vi "Overlay Results.vi"(5 "Name":string, 7 "Overlay Setup":T1, 8 "error in (no error)":errorcluster, 9 "Matches (pixels)":T2(array[cluster]) {"Bounding Box"."y" format="%.2f"; "Bounding Box"."x" format="%.2f"; "Position"."y" format="%.2f"; "Position"."x" format="%.2f"; "Score" format="%.2f"; "Scale" format="%.2f"; "Angle" format="%.2f"}, 10 "Search Area":T3 {"Contours"."Type" items=["No Selection", "Point", "Line", "Rectangle", "Oval", "Polygon", "Free", "Annulus", "Unused2", "Unused3", "Broken Line", "Free Hand Line", "Rotated Rectangle"]}, 11 "Image In":T4) -> (0 "error out":errorcluster, 2 "Elapsed Time (ms)":u32, 3 "Image Out":T4)   [LabVIEW 2017]
uses:
  <vilib>/vision/Image Controls.llb/IMAQ Image.ctl
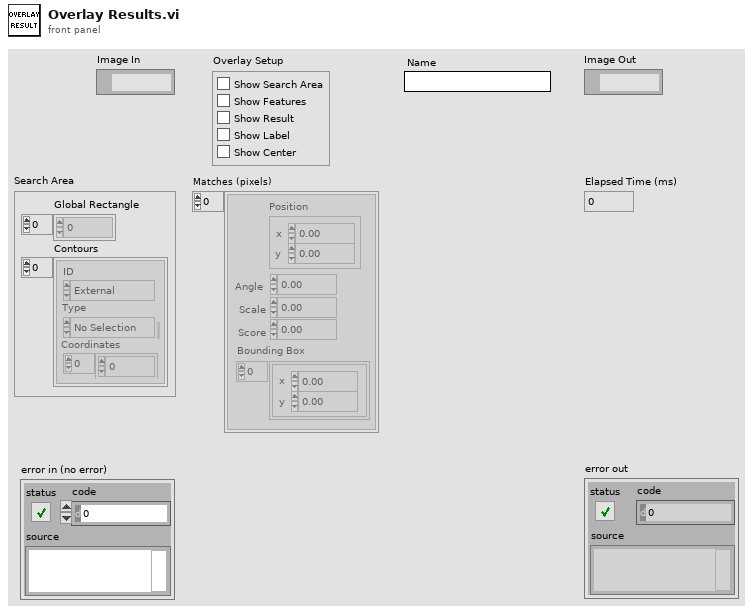
[diagram p1: front panel]
types:
  T1 = cluster{"Show Search Area":bool, "Show Features":bool, "Show Result":bool, "Show Label":bool, "Show Center":bool}
  T2 = cluster{"Position":cluster{"x":sgl, "y":sgl}, "Angle":sgl, "Scale":sgl, "Score":sgl, "Bounding Box":cluster{"x":sgl, "y":sgl}[]}[]
  T3 = cluster{"Global Rectangle":i32[], "Contours":cluster{"ID":enum32{"External", "Internal"}, "Type":u32, "Coordinates":i32[]}[]}
  T4 = typedef "IMAQ Image.ctl" = refnum<image>
  T5 = cluster{"Image":T4, "Search Area":cluster{"Global Rectangle":i32[], "Contours":cluster{"ID":enum32{"External", "Internal"}, "Type":u32, "Coordinates":i32[]}[]}, "Matches (pixels)":cluster{"Position":cluster{"x":sgl, "y":sgl}, "Angle":sgl, "Scale":sgl, "Score":sgl, "Bounding Box":cluster{"x":sgl, "y":sgl}[]}[], "Setup":cluster{"Show Search Area":bool, "Show Features":bool, "Show Result":bool, "Show Label":bool, "Show Center":bool}, "start time":u32, "Name":string}
  T6 = cluster{"Desired Font (Application)":enum16{"User-specified Font", "Application Font", "System Font", "Dialog Font"}, "[User-specified Font]":cluster{"Font Name":string, "Size":i16, "Strikeout?":bool, "Italic?":bool, "Underline?":bool, "Outline?":bool, "Shadow?":bool, "Bold?":bool, "Rotation Angle":dbl}, "Horizontal Alignment":i16, "Vertical Alignment":i16}
  T7 = cluster{"ID":enum32{"External", "Internal"}, "Type":u32, "Coordinates":i32[]}[]
  T8 = cluster{"ID":enum32{"External", "Internal"}, "Type":u32, "Coordinates":i32[]}
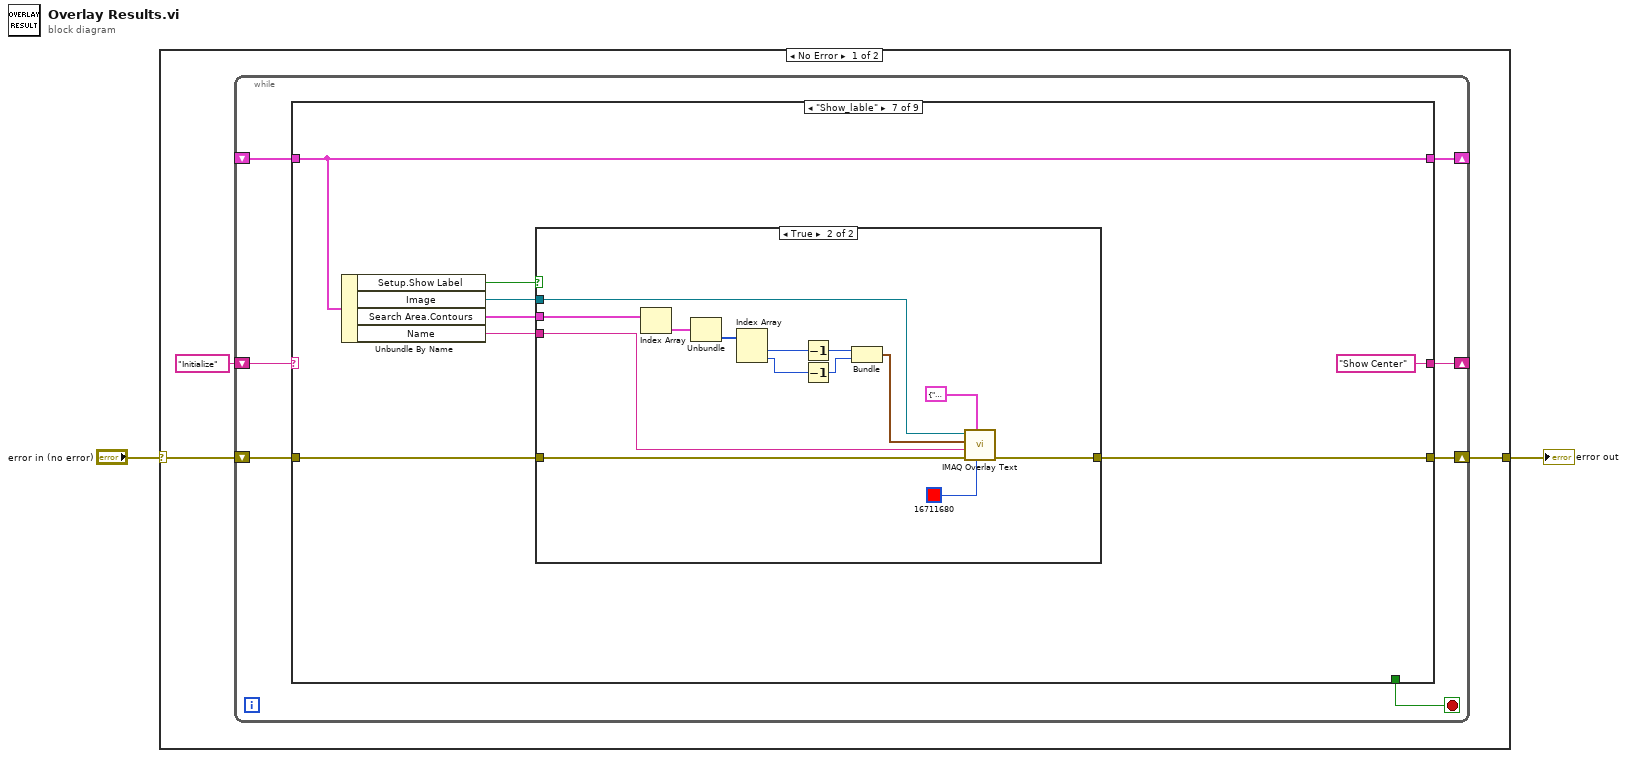
[diagram p0: block diagram]
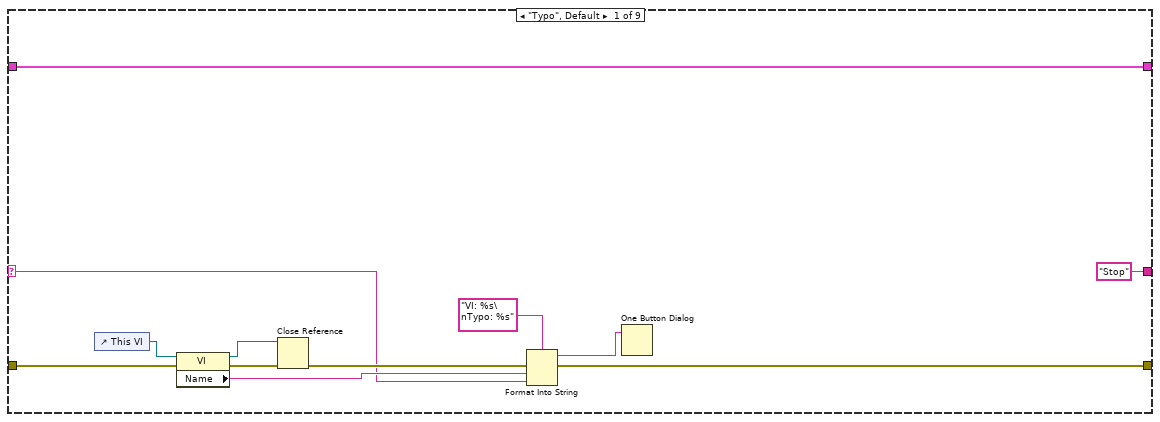
[diagram p2: hidden frame]
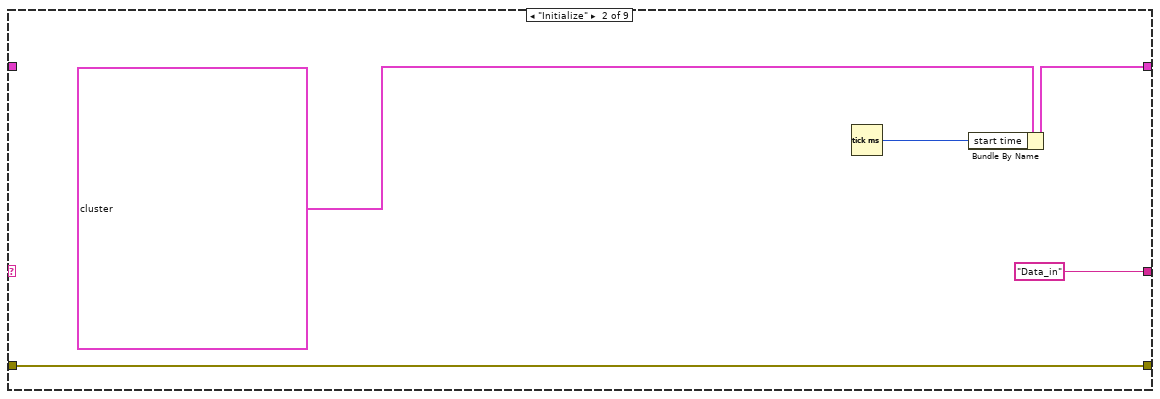
[diagram p3: hidden frame]
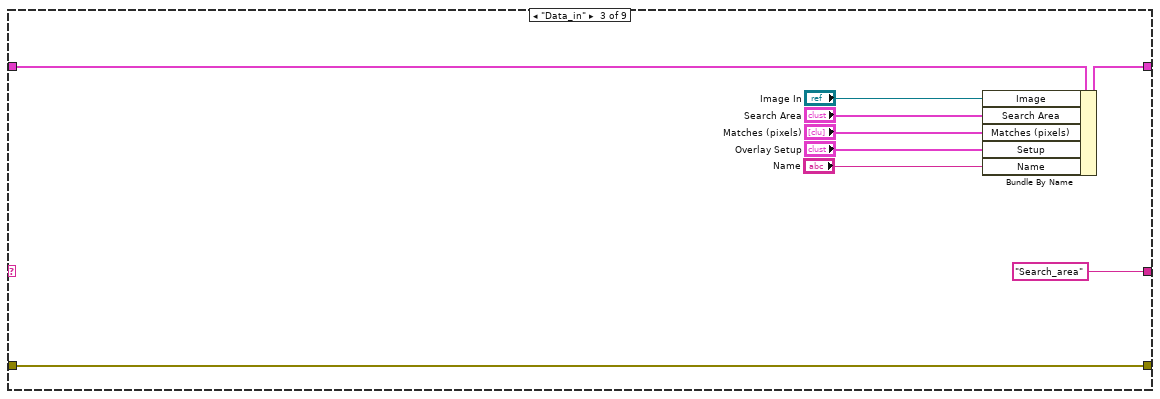
[diagram p4: hidden frame]
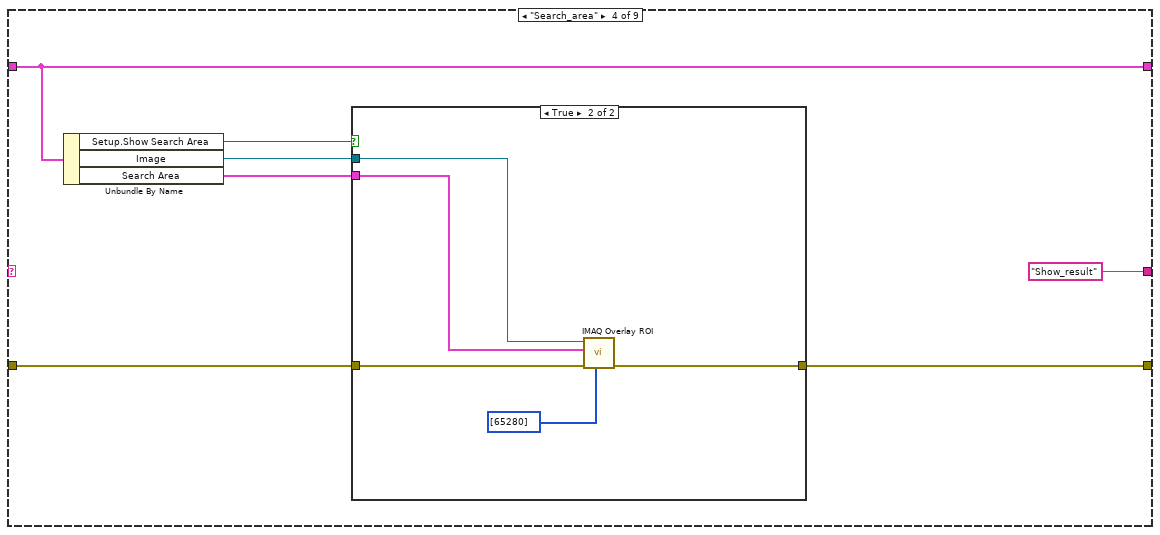
[diagram p5: hidden frame]
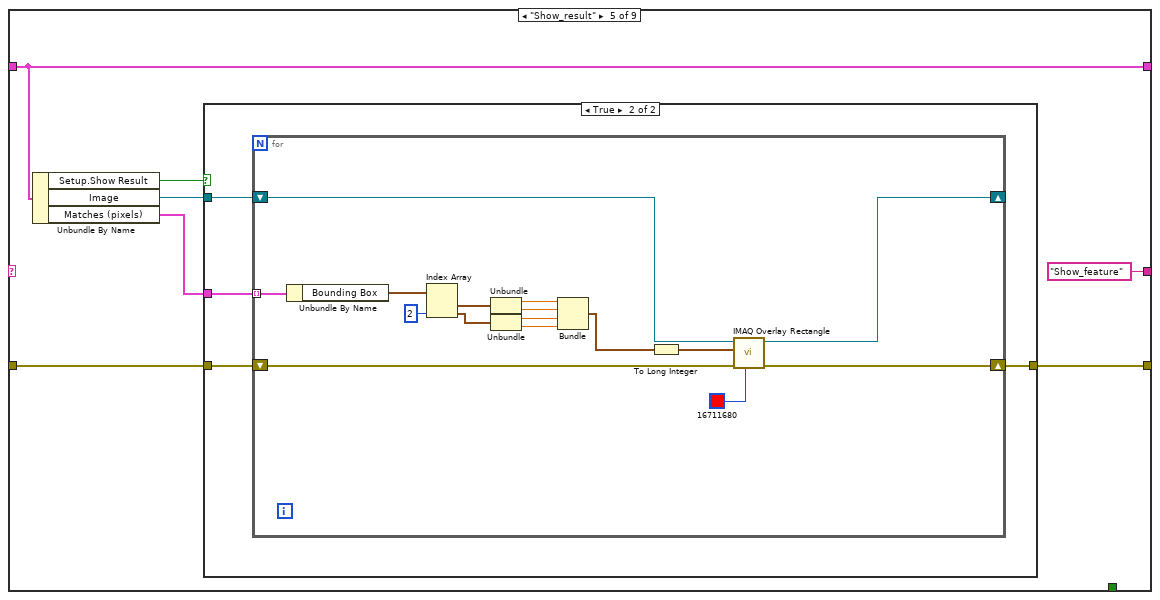
[diagram p7: hidden frame]
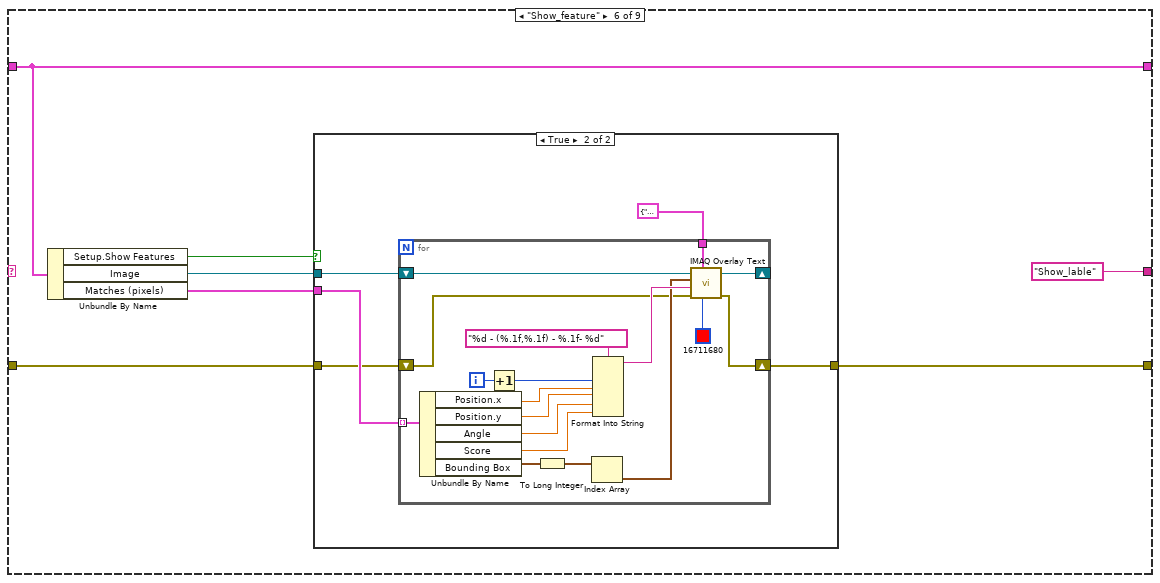
[diagram p9: hidden frame]
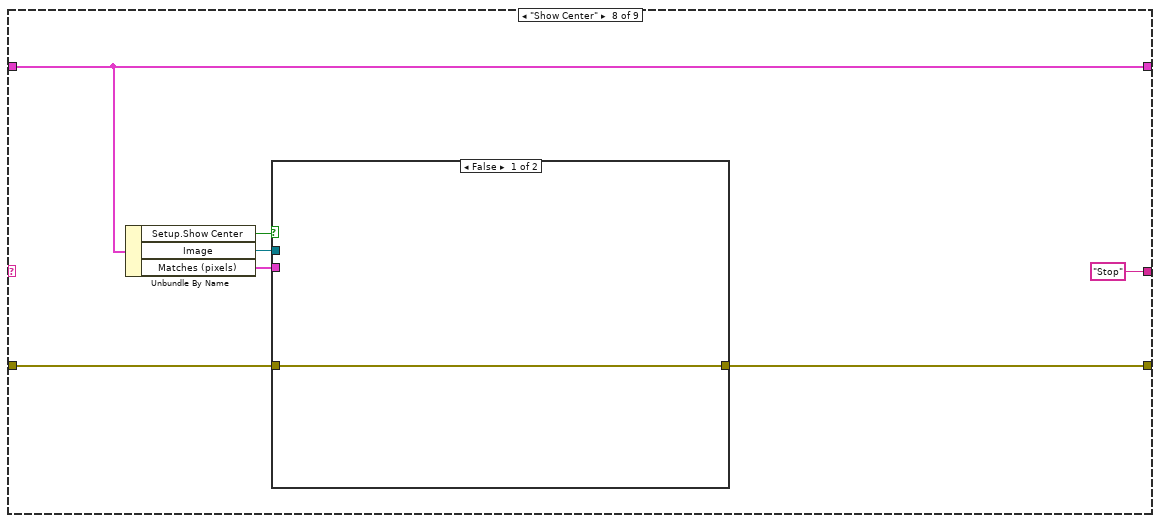
[diagram p12: hidden frame]
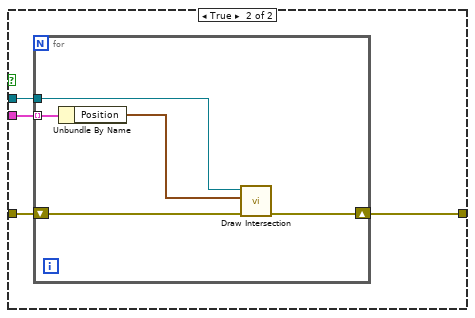
[diagram p13: hidden frame]
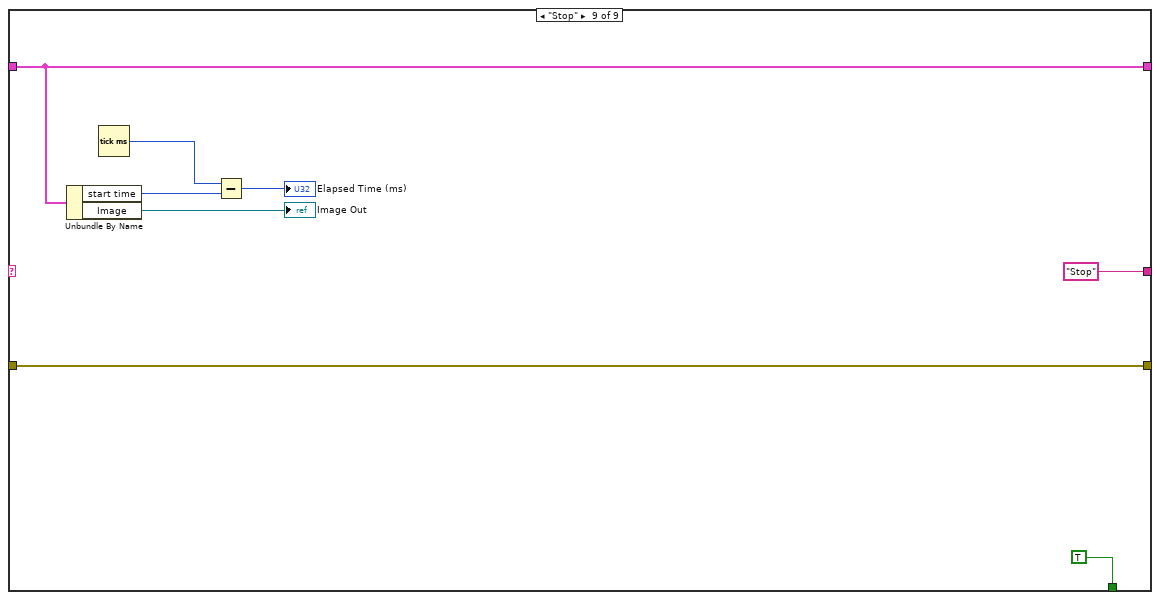
[diagram p14: hidden frame]
diagram:
  n1 = case shown="No Error" "error in (no error)" {
    selector: "error in (no error)" -> [w5 w159]
    tunnel: [w4 w159] -> w1
    frame No Error {
      n2 = while {
        shift-right: [w10] -> w4
        shift-left: w5 -> [w12]
        shift-right: [w7] -> _
        shift-left: "Initialize" -> [w11]
        shift-right: [w9] -> _
        shift-left: _ -> [w8]
        stop <- w6 stop-if-true
        n3 = case shown="\"Show_lable\"" w11 {
          selector: w11 -> [w15 _ _ _ _ _ _ _ _]
          tunnel: w12 -> [w23 w29 w32 w45 w55 w82 w116 w140 w158]
          tunnel: [w17 w29 w32 w44 w54 w81 w115 w139 w158] -> w10
          tunnel: [w24 w26 w37 w43 w58 w86 w118 w137 w155] -> w9
          tunnel: w8 -> [w24 _ w38 w43 w58 w86 w118 w137 w155]
          tunnel: ["Stop" "Data_in" "Search_area" "Show_result" "Show_feature" "Show_lable" "Show Center" "Stop" "Stop"] -> w7
          tunnel: [_ _ _ _ _ _ _ _ TRUE] -> w6
          frame "Typo", Default {
            n4 = control-ref of="This VI"() -> (w20:refnum<vi>)
            n5 = property class="VI"(reference=w20, error in=w23) -> (reference out=w18:refnum<vi>, error out=w21:errorcluster, "Name"=w16:string)
            n6 = Close Reference(reference=w18, error in (no error)=w21) -> (error out=w19:errorcluster)
            n7 = Format Into String(format string="VI: %s\nTypo: %s", error in=w19, w16, w15) -> (resulting string=w13:string, error out=w17:errorcluster)  [unwired: 1 in]
            n8 = One Button Dialog(message=w13) -> ()  [unwired: 1 in, 1 out]
          }
          frame "Initialize" {
            n9 = Tick Count (ms)() -> (millisecond timer value=w25:u32)
            n10 = Bundle By Name(cluster=T5 {"Image"=refnum, "Search Area"={"Global Rectangle"=[], "Contours"=[]}, "Matches (pixels)"=[], "Setup"={"Show Search Area"=FALSE, "Show Features"=FALSE, "Show Result"=FALSE, "Show Label"=FALSE, "Show Center"=FALSE}, "start time"=0, "Name"=""}, "start time"=w25) -> (w26:T5)
          }
          frame "Data_in" {
            n11 = Bundle By Name(cluster=w38, "Image"="Image In", "Search Area"="Search Area", "Matches (pixels)"="Matches (pixels)", "Setup"="Overlay Setup", "Name"="Name") -> (w37:T5)
          }
          frame "Search_area" {
            n12 = Unbundle By Name(w43) -> ("Setup.Show Search Area"=w42:bool, "Image"=w41:T4, "Search Area"=w40:T3)
            n13 = case shown="True" w42 {
              tunnel: w41 -> [_ w51]
              tunnel: w40 -> [_ w50]
              tunnel: w45 -> [w46 w49]
              tunnel: [w46 w48] -> w44
              frame False {
              }
              frame True {
                n14 = call "IMAQ Overlay ROI"("Colors (Green)"=u32[] [65280], "error in (no error)"=w49, "ROI Descriptor"=w50, "Image"=w51) -> ("error out"=w48:errorcluster)  [unwired: 6 in, 1 out]
              }
            }
          }
          frame "Show_result" {
            n15 = Unbundle By Name(w58) -> ("Setup.Show Result"=w53:bool, "Image"=w56:T4, "Matches (pixels)"=w57:T2)
            n16 = case shown="True" w53 {
              tunnel: w56 -> [_ w63]
              tunnel: w57 -> [_ w62]
              tunnel: w55 -> [w59 w61]
              tunnel: [w59 w60] -> w54
              frame False {
              }
              frame True {
                n17 = for {
                  shift-right: [w77] -> _
                  shift-left: w63 -> [w78]
                  tunnel: w62 -> [w79] mode=indexing
                  shift-right: [w75] -> w60
                  shift-left: w61 -> [w76]
                  n18 = Unbundle By Name(w79) -> ("Bounding Box"=w73:cluster{"x":sgl, "y":sgl}[])
                  n19 = Index Array(array=w73, index #2=2 ("index")) -> (element #1=w71:cluster{"x":sgl, "y":sgl}, element #2=w70:cluster{"x":sgl, "y":sgl})  [unwired: 1 in]
                  n20 = Unbundle(w71) -> ("x"=w69:sgl, "y"=w68:sgl)
                  n21 = Unbundle(w70) -> ("x"=w67:sgl, "y"=w66:sgl)
                  n22 = Bundle("x"=w69, "y"=w68, "x"=w67, "y"=w66) -> (w65:cluster{"x":sgl, "y":sgl, "x":sgl, "y":sgl})  [unwired: 1 in]
                  n23 = To Long Integer(number=w65) -> (32bit integer=w64:cluster{"x":i32, "y":i32, "x":i32, "y":i32})
                  n24 = call "IMAQ Overlay Rectangle"("Color"=u32 16711680, "error in (no error)"=w76, "Rectangle"=w64, "Image"=w78) -> ("error out"=w75:errorcluster, "Image Out"=w77:T4)  [unwired: 6 in]
                }
              }
            }
          }
          frame "Show_feature" {
            n25 = Unbundle By Name(w86) -> ("Setup.Show Features"=w83:bool, "Image"=w85:T4, "Matches (pixels)"=w84:T2)
            n26 = case shown="True" w83 {
              tunnel: w84 -> [_ w92]
              tunnel: w85 -> [_ w91]
              tunnel: w82 -> [w87 w89]
              tunnel: [w87 w88] -> w81
              frame False {
              }
              frame True {
                n27 = for {
                  shift-right: [w108] -> _
                  shift-left: w91 -> [w109]
                  tunnel: w92 -> [w110] mode=indexing
                  tunnel: T6 {"Desired Font (Application)"=enum."User-specified Font", "[User-specified Font]"={"Font Name"="NI Vision", "Size"=13, "Strikeout?"=FALSE, "Italic?"=FALSE, "Underline?"=FALSE, "Outline?"=FALSE, "Shadow?"=FALSE, "Bold?"=FALSE, "Rotation Angle"=0.0}, "Horizontal Alignment"=0, "Vertical Alignment"=0} ("Overlay Font Style") -> [w95]
                  shift-right: [w93] -> w88
                  shift-left: w89 -> [w94]
                  i -> [w106]
                  n28 = Unbundle By Name(w110) -> ("Position.x"=w103:sgl, "Position.y"=w102:sgl, "Angle"=w101:sgl, "Score"=w100:sgl, "Bounding Box"=w105:cluster{"x":sgl, "y":sgl}[])
                  n29 = Increment(x=w106) -> (x+1=w104:i32)
                  n30 = To Long Integer(number=w105) -> (32bit integer=w97:cluster{"x":i32, "y":i32}[])
                  n31 = Index Array(array=w97) -> (element=w96:cluster{"x":i32, "y":i32})  [unwired: 1 in]
                  n32 = Format Into String(format string="%d - (%.1f,%.1f) - %.1f- %d" ("Result String"), w104, w103, w102, w101, w100) -> (resulting string=w99:string)  [unwired: 2 in, 1 out]
                  n33 = call "IMAQ Overlay Text"("Text Color (black)"=u32 16711680, "Font, Size & Style"=w95, "error in (no error)"=w94, "String"=w99, "Origin"=w96, "Image"=w109) -> ("error out"=w93:errorcluster, "Image Out"=w108:T4)  [unwired: 4 in]
                }
              }
            }
          }
          frame "Show_lable" {
            n34 = Unbundle By Name(w118) -> ("Setup.Show Label"=w113:bool, "Image"=w117:T4, "Search Area.Contours"=w114:T7, "Name"=w111:string)
            n35 = case shown="True" w113 {
              tunnel: w117 -> [_ w133]
              tunnel: w116 -> [w119 w132]
              tunnel: [w119 w131] -> w115
              tunnel: w114 -> [_ w129]
              tunnel: w111 -> [_ w120]
              frame False {
              }
              frame True {
                n36 = Index Array(array=w129) -> (element=w128:T8)  [unwired: 1 in]
                n37 = Unbundle(w128) -> ("Coordinates"=w127:i32[])  [unwired: 2 out]
                n38 = Index Array(array=w127) -> (element #1=w126:i32, element #2=w125:i32)  [unwired: 2 in]
                n39 = Decrement(x=w126) -> (x-1=w124:i32)
                n40 = Decrement(x=w125) -> (x-1=w123:i32)
                n41 = Bundle(w124, w123) -> (w122:cluster{i32, i32})  [unwired: 1 in]
                n42 = call "IMAQ Overlay Text"("Text Color (black)"=u32 16711680, "Font, Size & Style"=T6 {"Desired Font (Application)"=enum."User-specified Font", "[User-specified Font]"={"Font Name"="NI Vision", "Size"=13, "Strikeout?"=FALSE, "Italic?"=FALSE, "Underline?"=FALSE, "Outline?"=FALSE, "Shadow?"=FALSE, "Bold?"=FALSE, "Rotation Angle"=0.0}, "Horizontal Alignment"=0, "Vertical Alignment"=0} ("Overlay Font Style"), "error in (no error)"=w132, "String"=w120, "Origin"=w122, "Image"=w133) -> ("error out"=w131:errorcluster)  [unwired: 4 in, 1 out]
              }
            }
          }
          frame "Show Center" {
            n43 = Unbundle By Name(w137) -> ("Setup.Show Center"=w134:bool, "Image"=w135:T4, "Matches (pixels)"=w136:T2)
            n44 = case shown="False" w134 {
              tunnel: w140 -> [w141 w145]
              tunnel: [w141 w144] -> w139
              tunnel: w136 -> [_ w143]
              tunnel: w135 -> [_ w142]
              frame False {
              }
              frame True {
                n45 = for {
                  shift-right: [w149] -> w144
                  shift-left: w145 -> [w150]
                  tunnel: w143 -> [w148] mode=indexing
                  tunnel: w142 -> [w146]
                  n46 = Unbundle By Name(w148) -> ("Position"=w147:cluster{"x":sgl, "y":sgl})
                  n47 = call "Draw Intersection.vi"("error in (no error)"=w150, "Intersection Point"=w147, "Refnum in"=w146) -> ("error out"=w149:errorcluster)  [unwired: 7 in, 1 out]
                }
              }
            }
          }
          frame "Stop" {
            n48 = Unbundle By Name(w155) -> ("start time"=w153:u32, "Image"=→"Image Out":T4)
            n49 = Tick Count (ms)() -> (millisecond timer value=w152:u32)
            n50 = Subtract(x=w152, y=w153) -> (x-y=→"Elapsed Time (ms)":u32)
          }
        }
      }
    }
    frame Error {
    }
  }
  "error out" <- w1
